vi "Synthetic_Jet_Initial.vi"() -> ()   [LabVIEW 2011]
uses:
  Globals/Meas_global.vi
  Acquisition/Data_Translation/DataTranslation_global.vi
panel:
  in  "Device Name":refnum<visa-resource-name>="USB0::0x0699::0x0347::C036837::INSTR"
  in  "Orifice diameter":dbl=0.0055
  out "Num of Blocks":i32=45
  in  "Dwell (ms)":u32=750
  in  "Samples per cycle":dbl=25.0
  in  "Amplitude Delta":dbl=3.0
  in  "Min Amplitude":dbl=3.0
  in  "Max Amplitude":dbl=6.0
  in  "Frequency Delta":dbl=10.0
  in  "Min Frequency":dbl=300.0
  in  "Max Frequency":dbl=1300.0
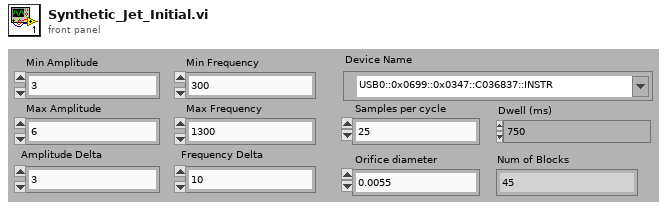
[diagram p1: front panel]
types:
  T1 = typedef "Post_Process.ctl" = enum16{"Take New Data", "Post Process Raw Data File"}
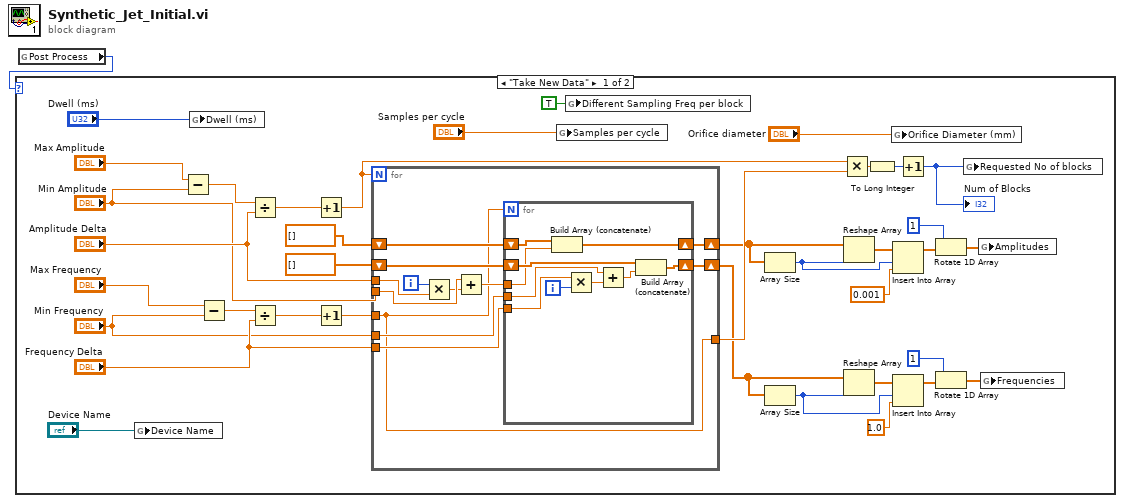
[diagram p0: block diagram]
diagram:
  n1 = global read "Meas_global.vi" "Post Process"() -> (w1:T1)
  n2 = case shown="\"Take New Data\"" w1 {
    frame "Take New Data" {
      n3 = global write "DataTranslation_global.vi" "Device Name"("Device Name") -> ()
      n4 = Subtract(x="Max Amplitude", y="Min Amplitude") -> (x-y=w37:dbl)
      n5 = global write "DataTranslation_global.vi" "Dwell (ms)"("Dwell (ms)") -> ()
      n6 = Subtract(x="Max Frequency", y="Min Frequency") -> (x-y=w36:dbl)
      n7 = Divide(x=w37, y="Amplitude Delta") -> (x/y=w34:dbl)
      n8 = Divide(x=w36, y="Frequency Delta") -> (x/y=w33:dbl)
      n9 = Increment(x=w34) -> (x+1=w27:dbl)
      n10 = Increment(x=w33) -> (x+1=w24:dbl)
      n11 = for {
        N: w27 -> [_]
        shift-right: [w50] -> w17
        shift-left: dbl[] [] -> [w49]
        shift-right: [w47] -> w6
        shift-left: dbl[] [] -> [w48]
        tunnel: w24 -> [w39]
        tunnel: "Amplitude Delta" -> [w46]
        tunnel: "Min Amplitude" -> [w42]
        tunnel: "Frequency Delta" -> [w43]
        tunnel: "Min Frequency" -> [w40]
        tunnel: [w39] -> w31
        i -> [w45]
        n12 = Multiply(x=w45, y=w46) -> (x*y=w41:dbl)
        n13 = Add(x=w42, y=w41) -> (x+y=w44:dbl)
        n14 = for {
          N: w39 -> [_]
          shift-right: [w60] -> w50
          shift-left: w49 -> [w59]
          shift-right: [w57] -> w47
          shift-left: w48 -> [w58]
          tunnel: w44 -> [w56]
          tunnel: w43 -> [w54]
          tunnel: w40 -> [w52]
          i -> [w55]
          n15 = Build Array (concatenate)(w59, w56) -> (w60:dbl[])
          n16 = Multiply(x=w54, y=w55) -> (x*y=w53:dbl)
          n17 = Add(x=w52, y=w53) -> (x+y=w51:dbl)
          n18 = Build Array (concatenate)(w58, w51) -> (w57:dbl[])
        }
      }
      n19 = global write "DataTranslation_global.vi" "Samples per cycle"("Samples per cycle") -> ()
      n20 = global write "DataTranslation_global.vi" "Different Sampling Freq per block"(TRUE ("Different Sampling Freq per block")) -> ()
      n21 = Array Size(array=w17) -> (size(s)=w5:i32)
      n22 = Array Size(array=w6) -> (size(s)=w4:i32)
      n23 = Multiply(x=w27, y=w31) -> (x*y=w20:dbl)
      n24 = Reshape Array(w17, w5) -> (w16:dbl[])
      n25 = Reshape Array(w6, w4) -> (w8:dbl[])
      n26 = To Long Integer(number=w20) -> (32bit integer=w19:i32)
      n27 = global write "DataTranslation_global.vi" "Orifice Diameter (mm)"("Orifice diameter") -> ()
      n28 = Insert Into Array(array=w16, index=w5, new element=0.001 ("new element/subarray")) -> (w14:dbl[])
      n29 = Insert Into Array(array=w8, index=w4, new element=1.0 ("new element/subarray")) -> (w10:dbl[])
      n30 = Increment(x=w19) -> (x+1=w18:i32)
      "Num of Blocks" <- w18
      n31 = Rotate 1D Array(1:w14, 2:1 ("n")) -> (0:w13:dbl[])
      n32 = Rotate 1D Array(1:w10, 2:1 ("n")) -> (0:w7:dbl[])
      n33 = global write "Meas_global.vi" "Requested No of blocks"(w18) -> ()
      n34 = global write "DataTranslation_global.vi" "Amplitudes"(w13) -> ()
      n35 = global write "DataTranslation_global.vi" "Frequencies"(w7) -> ()
    }
    frame "Post Process Raw Data File" {
    }
  }
